vi "бегущая лампочка.vi"() -> ()   [LabVIEW 2017]
panel:
  in  "stop":bool
  out "array":bool[](array[boolean])
  in  "Wait":dbl
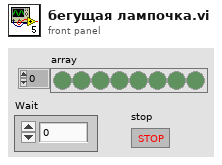
[diagram p1: front panel]
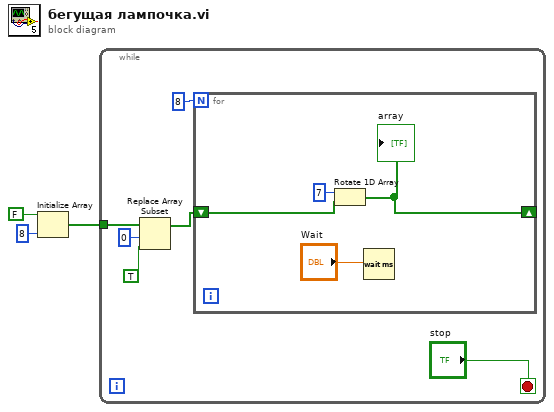
[diagram p0: block diagram]
diagram:
  n1 = Initialize Array(FALSE, 8 ("dimension size")) -> (w1:bool[])
  n2 = while {
    tunnel: w1 -> [w7]
    stop <- "stop" stop-if-true
    n3 = Replace Array Subset(array=w7, new element=TRUE, index=0) -> (w8:bool[])
    n4 = for {
      N: 8 -> [_]
      shift-right: [w10] -> _
      shift-left: w8 -> [w12]
      n5 = Rotate 1D Array(1:w12, 2:7 ("n")) -> (0:w10:bool[])
      "array" <- w10
      n6 = Wait (ms)(milliseconds to wait="Wait") -> ()  [unwired: 1 out]
    }
  }
